vi "Timer Count 2 with Error Handling.vi"(6 "Reset":bool, 8 "error in (no error)":errorcluster, 11 "Timeout (ms)":u32) -> (0 "error out":errorcluster, 1 "Elapsed Time(s)":dbl, 2 "Elapsed Time (ms)":u32, 3 "Timer Elapsed?":bool)   [LabVIEW 2014, in "Utilities.lvlib"]
uses:
  Utilities.lvlib
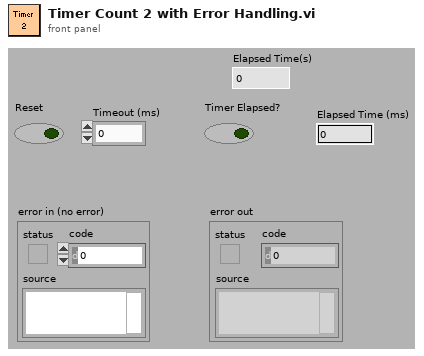
[diagram p1: front panel]
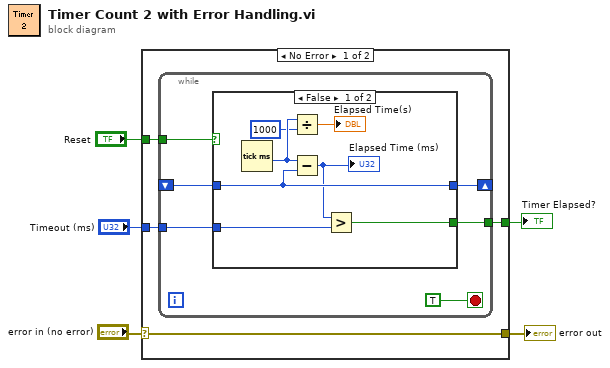
[diagram p0: block diagram]
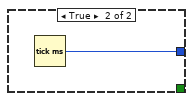
[diagram p2: hidden frame]
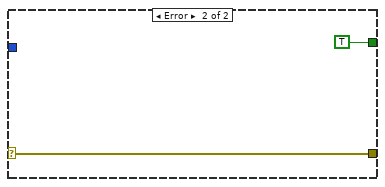
[diagram p3: hidden frame]
diagram:
  n1 = case shown="No Error" "error in (no error)" {
    selector: "error in (no error)" -> [w9 w25]
    tunnel: [w9 w25] -> w4
    tunnel: "Reset" -> [w8 _]
    tunnel: "Timeout (ms)" -> [w7 _]
    tunnel: [w6 TRUE] -> w1
    frame No Error {
      n2 = while {
        shift-right: [w14] -> _
        shift-left: _ -> [w12]
        tunnel: w8 -> [w13]
        tunnel: w7 -> [w11]
        tunnel: [w10] -> w6
        stop <- TRUE stop-if-true
        n3 = case shown="False" w13 {
          tunnel: [w22 w23] -> w14
          tunnel: w12 -> [w22 _]
          tunnel: w11 -> [w20 _]
          tunnel: [w19 _] -> w10
          frame False {
            n4 = Tick Count (ms)() -> (millisecond timer value=w18:u32)
            n5 = Divide(x=w18, y=u32 1000) -> (x/y=→"Elapsed Time(s)":dbl)
            n6 = Subtract(x=w18, y=w22) -> (x-y=w21:u32)
            "Elapsed Time (ms)" <- w21
            n7 = Greater?(x=w21, y=w20) -> (0:w19:bool)
          }
          frame True {
            n8 = Tick Count (ms)() -> (millisecond timer value=w23:u32)
          }
        }
      }
    }
    frame Error {
    }
  }
  "error out" <- w4
  "Timer Elapsed?" <- w1
